vi "GetTypedConfiguration.vi"(6 "Strict type matching? (F)":bool, 8 "error in (no error)":errorcluster, 9 "Name (empty: value name)":string, 10 "Default value":variant, 11 "SMO":refnum<class "SMO.lvclass">) -> (0 "error out":errorcluster, 1 "All Found":bool, 2 "Variant":variant, 3 "SMO out":refnum<class "SMO.lvclass">, 4 "Any Found":bool)   [LabVIEW 2013, in "SMO.lvclass"]
uses:
  SMO.lvclass
  Support/Attribute.Config/Attribute.Config.lvclass
panel:
  # "For instructions on how to use the JKI State Machine Objects, examples and video tutorials, visit:\nhttp://jki.net/state-machine-objects/\n\nJKI State Machine Objects™\nhttp://jki.net/state-machine-objects/\nCopyright (C) 2005-2015, JKI <info@jki.net>\nALL RIGHTS RESERVED"
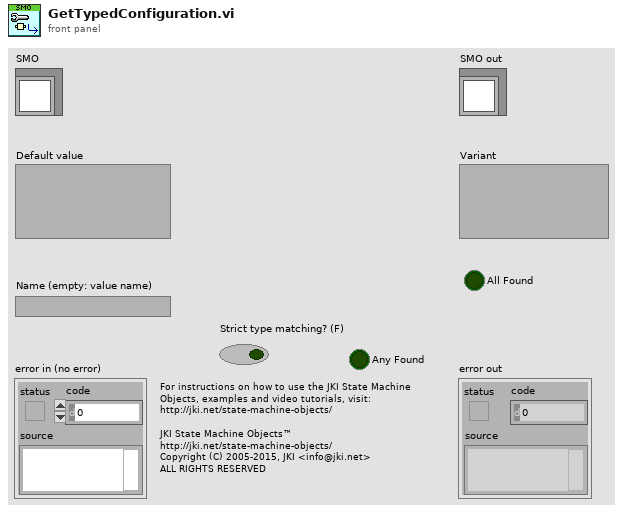
[diagram p1: front panel]
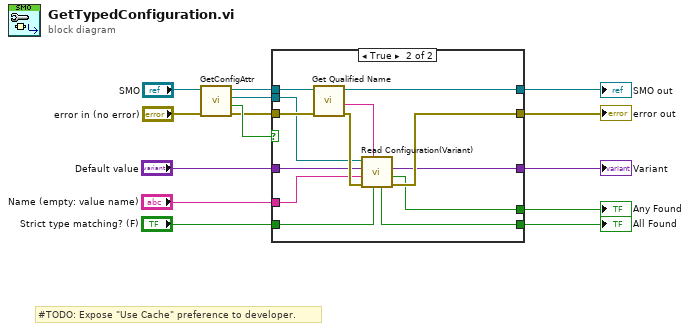
[diagram p0: block diagram]
diagram:
  # "#TODO: Expose \"Use Cache\" preference to developer."
  n1 = call "GetConfigAttr.vi"("error in (no error)"="error in (no error)", "SMO in"="SMO") -> ("error out"=w11:errorcluster, "found"=w13:bool, "Attribute.Config"=w12:refnum<class "Attribute.Config.lvclass">, "SMO out"=w14:refnum<class "SMO.lvclass">)  [unwired: 6 in]
  n2 = case shown="True" w13 {
    tunnel: w12 -> [_ w25]
    tunnel: w14 -> [w17 w30]
    tunnel: [w17 w28] -> w8
    tunnel: w11 -> [w16 w29]
    tunnel: [w16 w24] -> w7
    tunnel: [w15 w23] -> w6
    tunnel: [_ w22] -> w5
    tunnel: [_ w21] -> w4
    tunnel: "Name (empty: value name)" -> [_ w20]
    tunnel: "Default value" -> [w15 w19]
    tunnel: "Strict type matching? (F)" -> [_ w18]
    frame False {
    }
    frame True {
      n3 = call "Get Qualified Name.vi"("error in (no error)"=w29, "SMO"=w30) -> ("error out"=w26:errorcluster, "Reserved Qualified Name"=w27:string, "SMO out"=w28:refnum<class "SMO.lvclass">)  [unwired: 6 in, 1 out]
      n4 = call-dynamic "Read Configuration(Variant).vi"("Strict type matching? (F)"=w18, "Qualified Name"=w27, "error in (no error)"=w26, "Name (empty: value name)"=w20, "Default value"=w19, "Attribute.Config in"=w25) -> ("error out"=w24:errorcluster, "any found?"=w22:bool, "Variant"=w23:variant, "all found?"=w21:bool)  [unwired: 1 in, 1 out]
    }
  }
  "error out" <- w7
  "SMO out" <- w8
  "Variant" <- w6
  "Any Found" <- w5
  "All Found" <- w4
